vi "SanboxEngine.vi"() -> ()   [LabVIEW 2019]
uses:
  MB_ENGINE_class/Settings.ctl
  MB_ENGINE_class/Engine State.ctl
  MB_ENGINE_class/Engine Alarms.ctl
  MB_ENGINE_class/cmd enum.ctl
  MB_ENGINE_class/Switch Rule and Polarity.ctl
  MB_ENGINE_class/Limits Status.ctl
  MB_ENGINE_class/MB_ENGINE.lvclass
  D:/H4000/src/modbus engine custom/MB_MODULE_class/MB_MODULE.lvclass
  c692f2ff-c127-45f2-9d9c-48a2783b0954.vi
  f16da7fa-9700-40bc-8ecd-e9dd1a78cfb3.vi
  <vilib>/NI/Modbus Library/API/Wrapper/Create TCP Master.vi
  <vilib>/NI/Modbus Library/API/Wrapper/API Main.lvlib
  MB_MODULE_class/MB_MODULE.lvclass
panel:
  out "Limits":T1
  out "Switch Rule and Polarity  2":T2
  in  "Switch Rule and Polarity":T2={"Switch Rule"=1, "Polarity, F - NO, T - NC"=TRUE}
  in  "SW":u16=2
  out "angle":dbl(graph)
  out "dt":u32
  in  "cluster 2":T3={"ACC Steps Per Sec^2"=50, "DEC Steps Per Sec^2"=50, "Min Velosity Step Per Sec"=50, "Max Velosity Step Per Sec"=100, "MicroStep"=16}
  out "Numeric":i32
  out "Raw":i32(graph)
  out "RAW Possition Chart":i32(graph)
  in  "Set":bool
  in  "cmd to write":T4 items=["0 Idle"=0, "1 GoTo Absolute Position"=1, "2 GoTo Relative"=2, "10 GoTo Home Position"=10, "11 Set Home Position"=11, "12 Set FindHome Mode"=12, "13 Reset FindHome Mode"=13, "14 Get FindHome State"=14, "20 Hard Stop"=20, "21 HiZ Stop"=21, "22 Soft Stop"=22, "30 Clear Fault"=30, "40 Encoder Set Home"=40, "70 Driver Init"=70]
  in  "ARG I32":i32
  in  "On":bool
  in  "stop":bool
  out "type":u16
  out "Alarms":T5
  out "Engine State":T6 items=["ACCELERATING", "DECELERATINGTOSTOP", "DECELERATING", "STEADY", "INDEX_ACCEL", "NDEX_RUN", "INDEX_DECEL", "INDEX_DWELL", "INACTIVE", "STANDBY", "STANDBYTOINACTIVE"]
  out "RAW Possition":i32
  out "cluster":T3
  out "error out":errorcluster
  # "+ close\n- open"
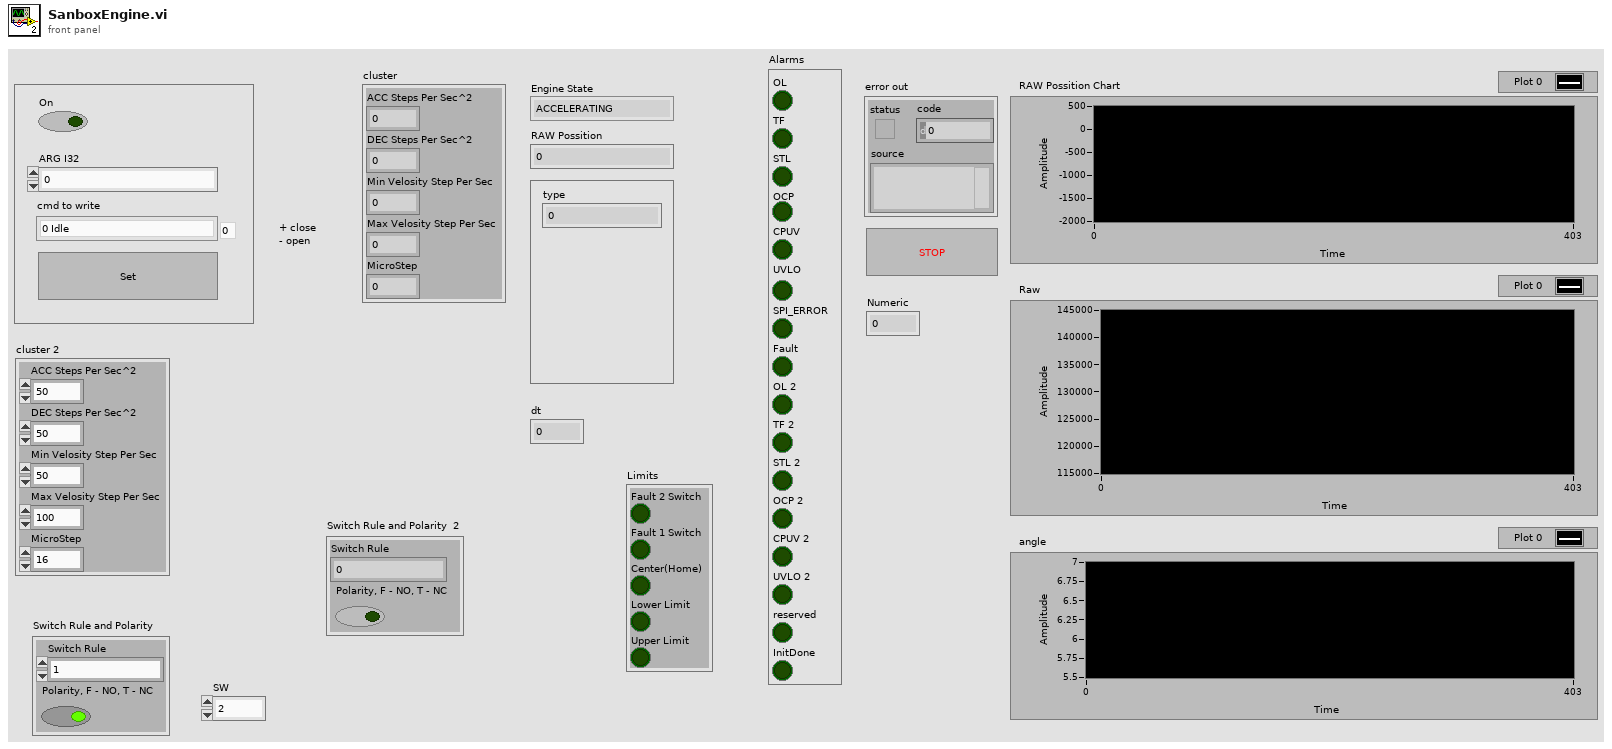
[diagram p1: front panel]
types:
  T1 = typedef "MB_ENGINE.lvclass/Limits Status.ctl" = cluster{"Fault 2 Switch":bool, "Fault 1 Switch":bool, "Center(Home)":bool, "Lower Limit":bool, "Upper Limit":bool}
  T2 = typedef "MB_ENGINE.lvclass/Switch Rule and Polarity.ctl" = cluster{"Switch Rule":u8, "Polarity, F - NO, T - NC":bool}
  T3 = typedef "MB_ENGINE.lvclass/Settings.ctl" = cluster{"ACC Steps Per Sec^2":u16, "DEC Steps Per Sec^2":u16, "Min Velosity Step Per Sec":u16, "Max Velosity Step Per Sec":u16, "MicroStep":u16}
  T4 = typedef "MB_ENGINE.lvclass/cmd enum.ctl" = u16
  T5 = typedef "MB_ENGINE.lvclass/Engine Alarms.ctl" = cluster{"OL":bool, "TF":bool, "STL":bool, "OCP":bool, "CPUV":bool, "UVLO":bool, "SPI_ERROR":bool, "Fault":bool, "OL 2":bool, "TF 2":bool, "STL 2":bool, "OCP 2":bool, "CPUV 2":bool, "UVLO 2":bool, "reserved":bool, "InitDone":bool}
  T6 = typedef "MB_ENGINE.lvclass/Engine State.ctl" = u16
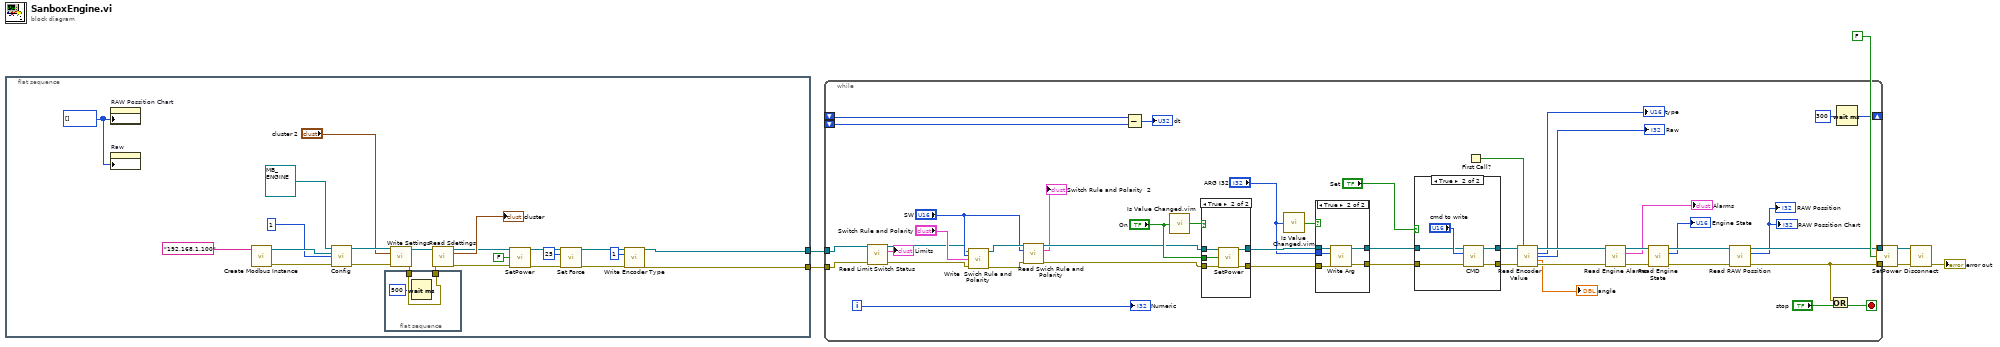
[diagram p0: block diagram]
diagram:
  n1 = flat-sequence {
    tunnel: [w10] -> w2
    tunnel: [w9] -> w1
    frame #0 {
      w13 = i32[] [] ("History Data")
      n2 = property on="RAW Possition Chart" class="WFChart (strict)"("History Data"=w13) -> ()  [unwired: 2 in, 2 out]
      n3 = property on="Raw" class="WFChart (strict)"("History Data"=w13) -> ()  [unwired: 2 in, 2 out]
      n4 = call-poly <vilib>:"Create Modbus Instance.vi"("address"="192.168.1.100") -> ("error out"=w29:errorcluster, "TCP master instance"=w31:refnum<class "Modbus Master.lvclass">)  [unwired: 9 in]
      n5 = call-dynamic "Config.vi"("class data in"=refnum<class "MB_ENGINE.lvclass"> refnum ("MB_ENGINE"), "modbus"=w31, "addres"=u16 1, "error in (no error)"=w29) -> ("class data out"=w26:refnum<class "MB_ENGINE.lvclass">, "error out"=w25:errorcluster)  [unwired: 10 in]
      n6 = flat-sequence {
        tunnel: [w34] -> w12
        tunnel: w11 -> [w34]
        frame #0 {
          n7 = Wait (ms)(milliseconds to wait=u32 500) -> ()  [unwired: 1 out]
        }
      }
      n8 = call-dynamic "Write Settings.vi"("class data in"=w26, "cluster"="cluster 2", "error in (no error)"=w25) -> ("class data out"=w23:refnum<class "MB_ENGINE.lvclass">, "error out"=w11:errorcluster)  [unwired: 11 in]
      n9 = call-dynamic "Read Sdettings.vi"("class data in"=w23, "error in (no error)"=w12) -> ("class data out"=w22:refnum<class "MB_ENGINE.lvclass">, "cluster"=→"cluster":T3, "error out"=w21:errorcluster)  [unwired: 11 in]
      n10 = call-dynamic "SetPower.vi"("class data in"=w22, "On"=FALSE, "error in (no error)"=w21) -> ("class data out"=w19:refnum<class "MB_ENGINE.lvclass">, "error out"=w18:errorcluster)  [unwired: 11 in]
      n11 = call-dynamic "Set Force.vi"("class data in"=w19, "percent"=u16 25, "error in (no error)"=w18) -> ("class data out"=w16:refnum<class "MB_ENGINE.lvclass">, "error out"=w15:errorcluster)  [unwired: 11 in]
      n12 = call-dynamic "Write Encoder Type.vi"("class data in"=w16, "U16"=u16 1, "error in (no error)"=w15) -> ("class data out"=w10:refnum<class "MB_ENGINE.lvclass">, "error out"=w9:errorcluster)  [unwired: 11 in]
    }
  }
  n13 = while {
    tunnel: [w74] -> w5
    tunnel: [w75] -> w6
    shift-right: [w60] -> _
    shift-left: _ -> [w59]
    shift-left: _ -> [w58]
    tunnel: w2 -> [w39]
    tunnel: w1 -> [w37]
    i -> [w62]
    stop <- w76 stop-if-true
    n14 = call-dynamic "Read Limit Switch Status.vi"("class data in"=w39, "error in (no error)"=w37) -> ("class data out"=w38:refnum<class "MB_ENGINE.lvclass">, "Limits"=→"Limits":T1, "error out"=w36:errorcluster)  [unwired: 11 in]
    n15 = call-dynamic "Write  Swich Rule and Polarity.vi"("class data in"=w38, "SW"="SW", "Switch Rule and Polarity"="Switch Rule and Polarity", "error in (no error)"=w36) -> ("class data out"=w42:refnum<class "MB_ENGINE.lvclass">, "error out"=w41:errorcluster)  [unwired: 10 in]
    n16 = call-dynamic "Read Swich Rule and Polarity.vi"("class data in"=w42, "SW"="SW", "error in (no error)"=w41) -> ("class data out"=w45:refnum<class "MB_ENGINE.lvclass">, "Switch Rule and Polarity"=→"Switch Rule and Polarity  2":T2, "error out"=w46:errorcluster)  [unwired: 10 in]
    n17 = Subtract(x=w59, y=w58) -> (x-y=→"dt":u32)
    n18 = call "Is Value Changed.vim"("value"="On") -> ("changed or first call?"=w72:bool)
    n19 = case shown="True" w72 {
      tunnel: w45 -> [w89 w94]
      tunnel: w46 -> [w88 w93]
      tunnel: "On" -> [_ w92]
      tunnel: [w89 w91] -> w71
      tunnel: [w88 w90] -> w70
      frame False {
      }
      frame True {
        n20 = call-dynamic "SetPower.vi"("class data in"=w94, "On"=w92, "error in (no error)"=w93) -> ("class data out"=w91:refnum<class "MB_ENGINE.lvclass">, "error out"=w90:errorcluster)  [unwired: 11 in]
      }
    }
    n21 = call "Is Value Changed.vim"("value"="ARG I32") -> ("changed or first call?"=w68:bool)
    n22 = case shown="True" w68 {
      tunnel: w71 -> [w96 w101]
      tunnel: w70 -> [w95 w100]
      tunnel: "ARG I32" -> [_ w99]
      tunnel: [w96 w98] -> w67
      tunnel: [w95 w97] -> w65
      frame False {
      }
      frame True {
        n23 = call-dynamic "Write Arg.vi"("class data in"=w101, "ARG U32"=w99, "error in (no error)"=w100) -> ("class data out"=w98:refnum<class "MB_ENGINE.lvclass">, "error out"=w97:errorcluster)  [unwired: 11 in]
      }
    }
    n24 = case shown="True" "Set" {
      tunnel: w67 -> [w81 w86]
      tunnel: [w81 w85] -> w66
      tunnel: w65 -> [w82 w84]
      tunnel: [w82 w83] -> w64
      frame False {
      }
      frame True {
        n25 = call-dynamic "CMD.vi"("class data in"=w86, "cmd to write"="cmd to write", "error in (no error)"=w84) -> ("class data out"=w85:refnum<class "MB_ENGINE.lvclass">, "error out"=w83:errorcluster)  [unwired: 11 in]
      }
    }
    n26 = First Call?() -> (First Call?: T/F=w54:bool)
    n27 = call-dynamic "Read Encoder Value.vi"("class data in"=w66, "init"=w54, "error in (no error)"=w64) -> ("class data out"=w80:refnum<class "MB_ENGINE.lvclass">, "type"=→"type":u16, "Encoder"=→"Raw":i32, "Angel (rad)"=→"angle":dbl, "error out"=w79:errorcluster)  [unwired: 8 in]
    n28 = call-dynamic "Read Engine Alarms.vi"("class data in"=w80, "error in (no error)"=w79) -> ("class data out"=w53:refnum<class "MB_ENGINE.lvclass">, "Alarms"=→"Alarms":T5, "error out"=w51:errorcluster)  [unwired: 11 in]
    n29 = call-dynamic "Read Engine State.vi"("class data in"=w53, "error in (no error)"=w51) -> ("class data out"=w52:refnum<class "MB_ENGINE.lvclass">, "Engine State"=→"Engine State":T6, "error out"=w50:errorcluster)  [unwired: 11 in]
    n30 = call-dynamic "Read RAW Possition.vi"("class data in"=w52, "error in (no error)"=w50) -> ("class data out"=w75:refnum<class "MB_ENGINE.lvclass">, "RAW Possition"=→"RAW Possition" →"RAW Possition Chart":i32, "error out"=w74:errorcluster)  [unwired: 11 in]
    n31 = Or(x=w74, y="stop") -> (x .or. y?=w76:bool)
    n32 = Wait (ms)(milliseconds to wait=u32 300) -> (millisecond timer value=w60:u32)
    "Numeric" <- w62
  }
  n33 = call-dynamic "SetPower.vi"("class data in"=w6, "On"=FALSE, "error in (no error)"=w5) -> ("class data out"=w3:refnum<class "MB_ENGINE.lvclass">, "error out"=w4:errorcluster)  [unwired: 11 in]
  n34 = call "Disconnect.vi"("MB_MODULE"=w3, "error in"=w4) -> ("error out"=→"error out":errorcluster)  [unwired: 13 in]
